vi "DSF.Engine.Execution.Transfer.RT FIFO.Create.vi"(8 "error in (no error)":errorcluster, 10 "r/w modes (polling, polling)":T2, 11 "size":u32) -> (0 "error out":errorcluster, 3 "Transfer FIFO":T1)   [LabVIEW 2016, in "DSF.Engine.lvlib" / "DSF.Engine.Execution.Transfer.lvclass"]
uses:
  DSF.Engine.Execution.Transfer.lvclass
  DSF.Engine.Execution.Transfer.RT FIFO Ref.ctl
  DSF.Engine.Execution.Transfer.RT FIFO Data.ctl
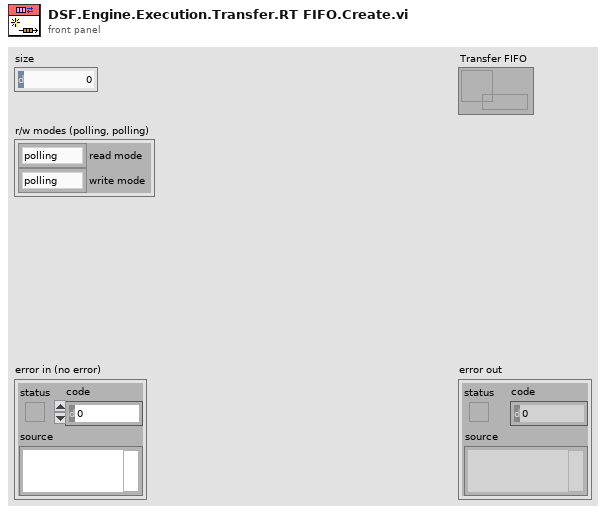
[diagram p1: front panel]
types:
  T1 = typedef "DSF.Engine.lvlib/DSF.Engine.Execution.Transfer.lvclass/DSF.Engine.Execution.Transfer.RT FIFO Ref.ctl" = refnum<k33>
  T2 = cluster{"read mode":enum16{"polling", "blocking"}, "write mode":enum16{"polling", "blocking"}}
  T3 = typedef "DSF.Engine.lvlib/DSF.Engine.Execution.Transfer.lvclass/DSF.Engine.Execution.Transfer.RT FIFO Data.ctl" = cluster{"ID":i32, "Buffer Descriptor":cluster{"address":u64, "size":u64}}
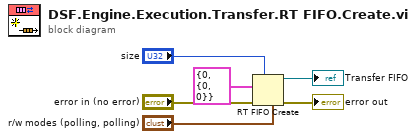
[diagram p0: block diagram]
diagram:
  n1 = RT FIFO Create(1:T3 {"ID"=0, "Buffer Descriptor"={"address"=0, "size"=0}} ("Transfer Data"), 3:"error in (no error)", 4:"size", 7:"r/w modes (polling, polling)") -> (8:→"Transfer FIFO":refnum<k33>, 11:→"error out":errorcluster)  [unwired: 4 in, 1 out]
